vi "History log.vi"(4 "Message":string="File is importing...", 7 "String IN":string) -> (3 "String OUT":string)   [LabVIEW 2017]
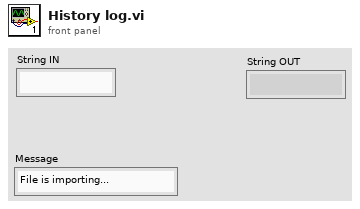
[diagram p1: front panel]
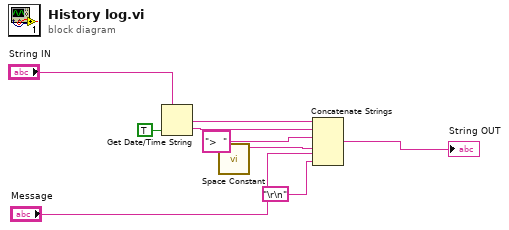
[diagram p0: block diagram]
diagram:
  n1 = Get Date/Time String(want seconds? (F)=TRUE ("초 보이기? (거짓)")) -> (time string=w6:string)  [unwired: 2 in, 1 out]
  n2 = call <vilib>:"Space Constant.vi"() -> ("String"=w4:string)
  n3 = Concatenate Strings("String IN", w6, ">  " ("문자열"), w4, "Message", "\r\n") -> (→"String OUT":string)
